vi "Robo Team Read INI.vi"() -> (0 "error out":errorcluster, 1 "Controller Log Path":string, 2 "Controller IP":string, 3 "Offset":T2, 5 "Controller Setup":T1={"Pitch Ratio"=1, "Roll Ratio"=1, "Yaw Ratio"=1, "Host IP"="", "Yaw Exist?"=FALSE, "Acceleration"=60000, "Hold Current"=5, "Run Current"=50, "Velocity"=10000, "Pitch Gain"=3000, "Roll Gain"=-3000, "Homing at Startup?"=FALSE, "Extended Logging"=FALSE} {"Yaw Ratio" min=1; "Roll Ratio" min=1; "Pitch Ratio" min=1})   [LabVIEW 2015]
uses:
  Robo Team Offset.ctl
  Robo Team Controller Setup.ctl
  <vilib>/Utility/config.llb/Read Key (Double).vi
  <vilib>/Utility/config.llb/Read Key (String).vi
  <vilib>/Utility/config.llb/Read Key (Boolean).vi
  <vilib>/Utility/config.llb/NI_LVConfig.lvlib
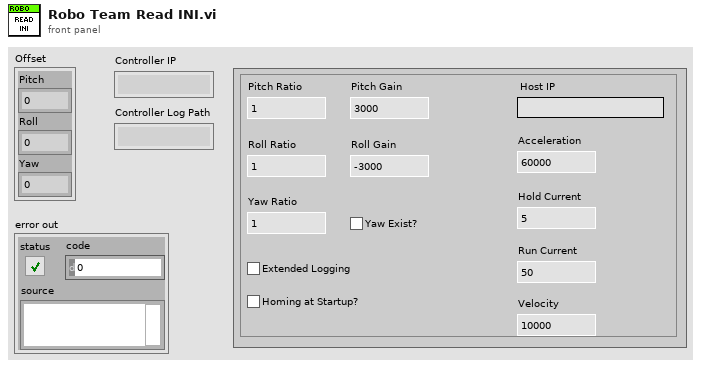
[diagram p1: front panel]
types:
  T1 = typedef "Robo Team Controller Setup.ctl" = cluster{"Pitch Ratio":i32, "Roll Ratio":i32, "Yaw Ratio":i32, "Host IP":string, "Yaw Exist?":bool, "Acceleration":i32, "Hold Current":i32, "Run Current":i32, "Velocity":i32, "Pitch Gain":i32, "Roll Gain":i32, "Homing at Startup?":bool, "Extended Logging":bool}
  T2 = typedef "Robo Team Offset.ctl" = cluster{"Pitch":dbl, "Roll":dbl, "Yaw":dbl}
  T3 = typedef "NI_LVConfig.lvlib/Config Data RefNum.ctl" = refnum<k1>
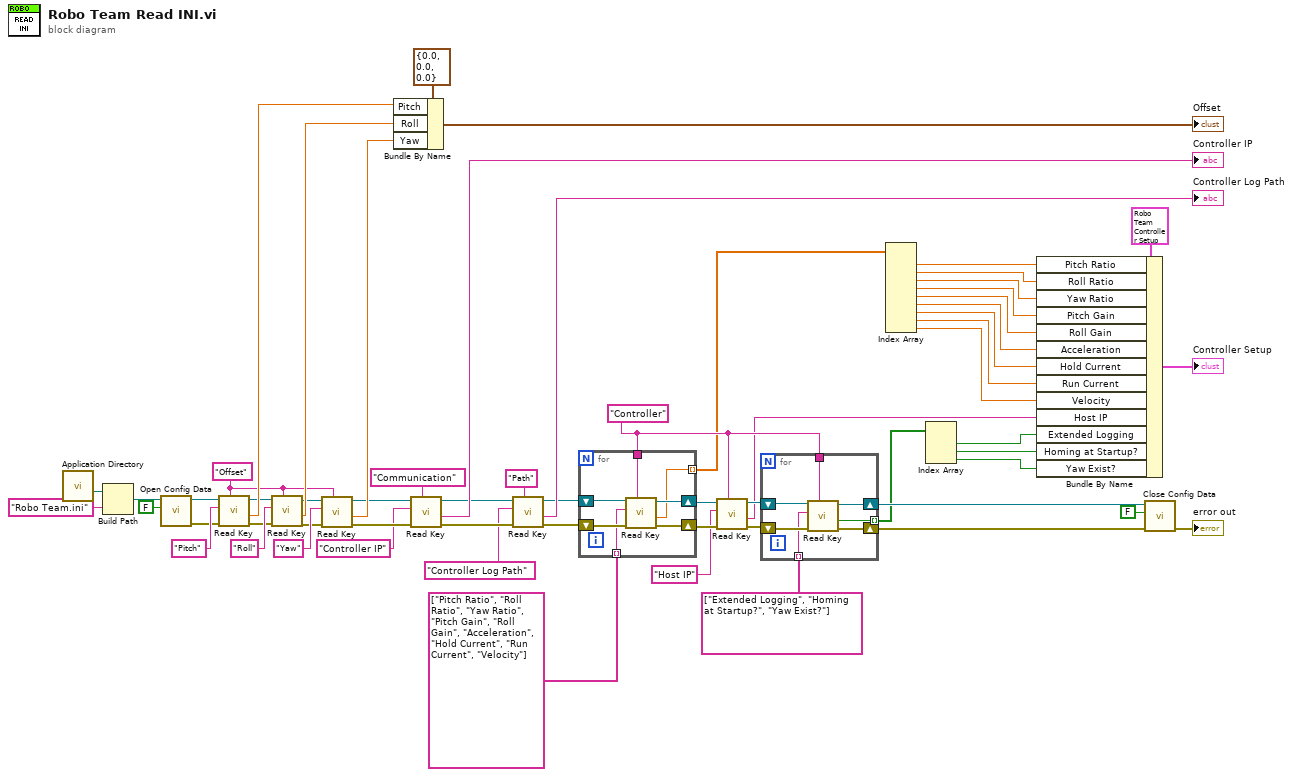
[diagram p0: block diagram]
diagram:
  w18 = "Controller" ("section")
  w51 = "Offset" ("section")
  n1 = call <vilib>:"Application Directory.vi"() -> ("Application Directory"=w40:path)
  n2 = Build Path(base path=w40, name or relative path="Robo Team.ini") -> (appended path=w42:path)
  n3 = call <vilib>:"Open Config Data.vi"("create file if necessary (T)"=FALSE, "configuration file path"=w42) -> ("error out"=w44:errorcluster, "refnum"=w45:T3)  [unwired: 7 in, 1 out]
  n4 = call-poly <vilib>:"Read Key.vi"("section"=w51, "error in (no error)"=w44, "key"="Pitch", "refnum"=w45) -> ("error out"=w47:errorcluster, "value"=w55:dbl, "refnum out"=w48:T3)  [unwired: 4 in, 1 out]
  n5 = call-poly <vilib>:"Read Key.vi"("section"=w51, "error in (no error)"=w47, "key"="Roll", "refnum"=w48) -> ("error out"=w49:errorcluster, "value"=w56:dbl, "refnum out"=w50:T3)  [unwired: 4 in, 1 out]
  n6 = call-poly <vilib>:"Read Key.vi"("section"=w51, "error in (no error)"=w49, "key"="Yaw", "refnum"=w50) -> ("error out"=w39:errorcluster, "value"=w57:dbl, "refnum out"=w35:T3)  [unwired: 4 in, 1 out]
  n7 = Bundle By Name(cluster=T2 {"Pitch"=0.0, "Roll"=0.0, "Yaw"=0.0}, "Pitch"=w55, "Roll"=w56, "Yaw"=w57) -> (→"Offset":T2)
  n8 = call-poly <vilib>:"Read Key.vi"("section"="Communication", "error in (no error)"=w39, "key"="Controller IP", "refnum"=w35) -> ("error out"=w34:errorcluster, "value"=→"Controller IP":string, "refnum out"=w33:T3)  [unwired: 4 in, 1 out]
  n9 = call-poly <vilib>:"Read Key.vi"("section"="Path", "error in (no error)"=w34, "key"="Controller Log Path", "refnum"=w33) -> ("error out"=w28:errorcluster, "value"=→"Controller Log Path":string, "refnum out"=w29:T3)  [unwired: 4 in, 1 out]
  n10 = for {
    tunnel: string[] ["Pitch Ratio", "Roll Ratio", "Yaw Ratio", "Pitch Gain", "Roll Gain", "Acceleration", "Hold Current", "Run Current", "Velocity"] -> [w65] mode=indexing
    shift-right: [w64] -> w25
    shift-left: w29 -> [w66]
    shift-right: [w63] -> w26
    shift-left: w28 -> [w67]
    tunnel: w18 -> [w62]
    tunnel: [w61] -> w15 mode=indexing
    n11 = call-poly <vilib>:"Read Key.vi"("section"=w62, "error in (no error)"=w67, "key"=w65, "refnum"=w66) -> ("error out"=w63:errorcluster, "value"=w61:dbl, "refnum out"=w64:T3)  [unwired: 4 in, 1 out]
  }
  n12 = call-poly <vilib>:"Read Key.vi"("section"=w18, "error in (no error)"=w26, "key"="Host IP", "refnum"=w25) -> ("error out"=w20:errorcluster, "value"=w5:string, "refnum out"=w21:T3)  [unwired: 4 in, 1 out]
  n13 = for {
    tunnel: string[] ["Extended Logging", "Homing at Startup?", "Yaw Exist?"] -> [w72] mode=indexing
    shift-right: [w71] -> w23
    shift-left: w21 -> [w73]
    shift-right: [w70] -> w22
    shift-left: w20 -> [w74]
    tunnel: w18 -> [w69]
    tunnel: [w68] -> w4 mode=indexing
    n14 = call-poly <vilib>:"Read Key.vi"("section"=w69, "error in (no error)"=w74, "key"=w72, "refnum"=w73) -> ("error out"=w70:errorcluster, "value"=w68:bool, "refnum out"=w71:T3)  [unwired: 4 in, 1 out]
  }
  n15 = Index Array(array=w15) -> (element #1=w14:dbl, element #2=w13:dbl, element #3=w12:dbl, element #4=w11:dbl, element #5=w10:dbl, element #6=w9:dbl, element #7=w8:dbl, element #8=w7:dbl, element #9=w6:dbl)  [unwired: 9 in]
  n16 = Index Array(array=w4) -> (element #1=w3:bool, element #2=w2:bool, element #3=w1:bool)  [unwired: 3 in]
  n17 = Bundle By Name(cluster=T1 {"Pitch Ratio"=1, "Roll Ratio"=1, "Yaw Ratio"=1, "Host IP"="", "Yaw Exist?"=FALSE, "Acceleration"=60000, "Hold Current"=5, "Run Current"=50, "Velocity"=10000, "Pitch Gain"=3000, "Roll Gain"=-3000, "Homing at Startup?"=FALSE, "Extended Logging"=FALSE} ("Controller Setup"), "Pitch Ratio"=w14, "Roll Ratio"=w13, "Yaw Ratio"=w12, "Pitch Gain"=w11, "Roll Gain"=w10, "Acceleration"=w9, "Hold Current"=w8, "Run Current"=w7, "Velocity"=w6, "Host IP"=w5, "Extended Logging"=w3, "Homing at Startup?"=w2, "Yaw Exist?"=w1) -> (→"Controller Setup":T1)
  n18 = call <vilib>:"Close Config Data.vi"("error in (no error)"=w22, "write file if changed (T)"=FALSE, "refnum"=w23) -> ("error out"=→"error out":errorcluster)  [unwired: 7 in, 1 out]
